vi "Init.vi"(8 "error in":errorcluster, 11 "Cell View Back Color Alternate in":refnum<class "Cell View Back Color Alternate.lvclass">) -> (0 "error out":errorcluster, 3 "Cell View Back Color Alternate out":refnum<class "Cell View Back Color Alternate.lvclass">)   [LabVIEW 2024]
uses:
  Cell View Back Color Alternate.lvclass/Cell View Back Color Alternate.ctl
  Cell View Back Color Alternate.lvclass
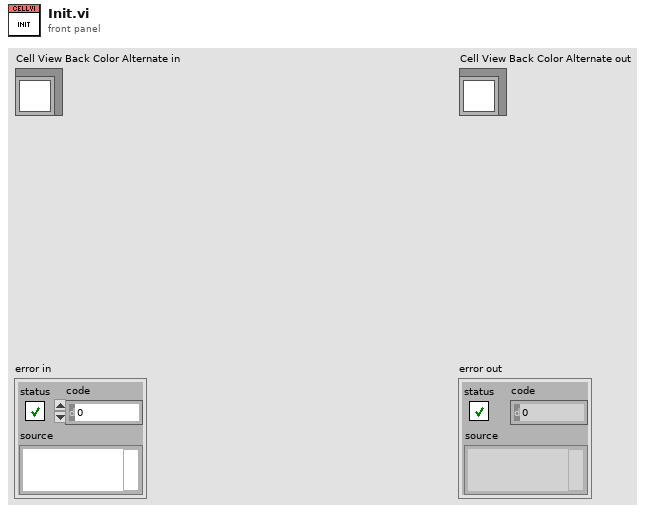
[diagram p1: front panel]
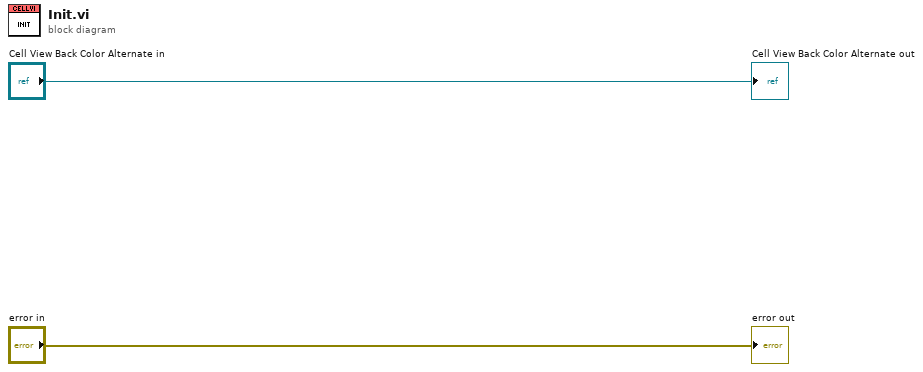
[diagram p0: block diagram]
diagram:
  "error out" <- "error in"
  "Cell View Back Color Alternate out" <- "Cell View Back Color Alternate in"
